vi "Set Sciscan Scope Image Averaging.vi"(8 "error in":errorcluster, 9 "Frames":i8, 10 "Average":u16(ring) items=["No Average", "Group Average", "Moving Average"], 11 "GFG Refnum":refnum<vi>) -> (0 "error out":errorcluster, 3 "GFG Refnum Out":refnum<vi>)   [LabVIEW 2012, in "Sciscan Scope Daemon.lvlib"]
uses:
  Sciscan Scope Daemon.lvlib
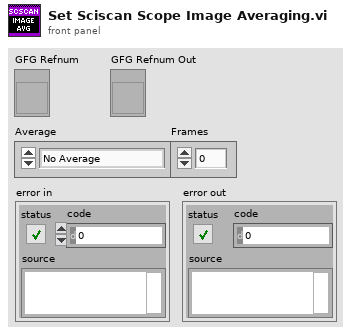
[diagram p1: front panel]
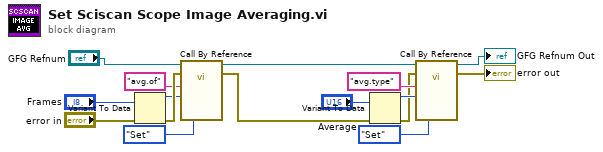
[diagram p0: block diagram]
diagram:
  n1 = Variant To Data(error in="error in", type="Frames", Variant="Frames") -> (data=w15:i8, error out=w16:errorcluster)
  n2 = call-by-ref "?"(reference="GFG Refnum", error in=w16, "Variable Name in"="avg.of", "Variant in"=w15, "Action"=enum16{"Init", "Set", "Get"}."Set") -> (reference out=w5:refnum<vi>, error out=w6:errorcluster)  [unwired: 10 in, 7 out]
  n3 = Variant To Data(error in=w6, type="Average", Variant="Average") -> (data=w8:u16, error out=w7:errorcluster)
  n4 = call-by-ref "?"(reference=w5, error in=w7, "Variable Name in"="avg.type", "Variant in"=w8, "Action"=enum16{"Init", "Set", "Get"}."Set") -> (reference out=→"GFG Refnum Out":refnum<vi>, error out=→"error out":errorcluster)  [unwired: 10 in, 7 out]
